vi "Smite - Simple.vi"() -> ()   [LabVIEW 2017]
doc: "A demonstration of smiting the zombie (enabled legacy code) at the grave (Diagram Disable Structure). This includes step-by-step instructions for enabling the Spirit (refactored) frame and disabling the Zombie (legacy) frame for the grave with one of two methods: shortcut menu plugin or Quick Drop shortcut plugin."
panel:
  out "Any?":bool
  in  "Input":bool[](array[boolean])=[FALSE, FALSE, FALSE, FALSE, TRUE, FALSE, FALSE]
  # "Overview: Demonstrates smiting (disabling) the legacy code that is currently enabled (zombie)\nInstructions:\n1. Run the VI\n2. Observe the value of the Any? indicator\n3. Uncheck the TRUE element in the Input array\n4. Run the VI\n5. Observe the value of the Any? indicator\n6. Switch to the block diagram and follow the instructions to use the refactored code"
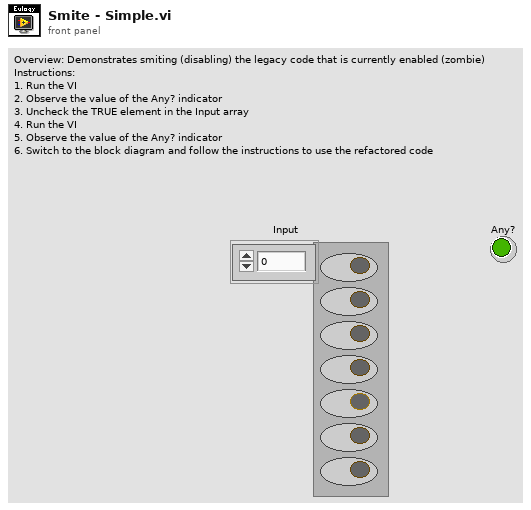
[diagram p1: front panel]
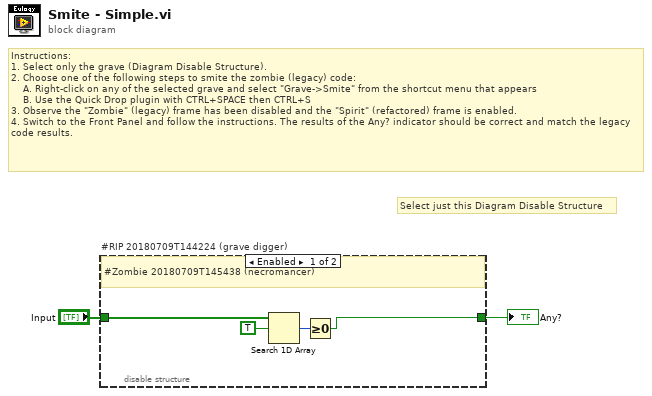
[diagram p0: block diagram]
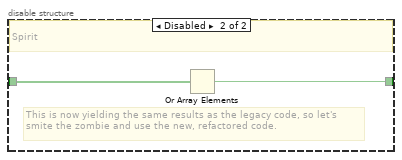
[diagram p2: hidden frame]
diagram:
  # "Select just this Diagram Disable Structure"
  # "Instructions:\n1. Select only the grave (Diagram Disable Structure).\n2. Choose one of the following steps to smite the zombie (legacy) code:\n    A. Right-click on any of the selected grave and select \"Grave->Smite\" from the shortcut menu that appears\n    B. Use the Quick Drop plugin with CTRL+SPACE then CTRL+S\n3. Observe the \"Zombie\" (legacy) frame has been disabled and the \"Spirit\" (refactored) frame is enabled.\n4. Switch to the Front Panel and follow the instructions. The results of the Any? indicator should be correct and match the legacy code results."
  n1 = disable-structure "#RIP 20180709T144224 (grave digger)" shown="Enabled" {
    disable-tunnel: "Input" -> [w6 w8]
    disable-tunnel: [w5 w7] -> w1
    frame Enabled {
      # "#Zombie 20180709T145438 (necromancer)"
      n2 = Search 1D Array(1D array=w6, element=TRUE) -> (index of element=w3:i32)  [unwired: 1 in]
      n3 = Greater Or Equal To 0?(x=w3) -> (x >= 0?=w5:bool)
    }
    frame Disabled {
      # "This is now yielding the same results as the legacy code, so let's smite the zombie and use the new, refactored code."
      # "Spirit"
      n4 = Or Array Elements(Boolean array=w8) -> (logical OR=w7:bool)
    }
  }
  "Any?" <- w1
